vi "Load DB Table.vi"(8 "error in (no error)":errorcluster, 10 "Calibration Mode":bool=TRUE, 11 "ENET in":refnum<class "ENET_BS120x.lvclass">) -> (0 "error out":errorcluster, 3 "ENET out":refnum<class "ENET_BS120x.lvclass">)   [LabVIEW 2021, in "BS120x Driver.lvlib" / "ENET_BS120x.lvclass"]
uses:
  ENET_BS120x.lvclass
  ENET_BS120x.lvclass/ENET_BS120x.ctl
  <resource>/objmgr/xnet.rc
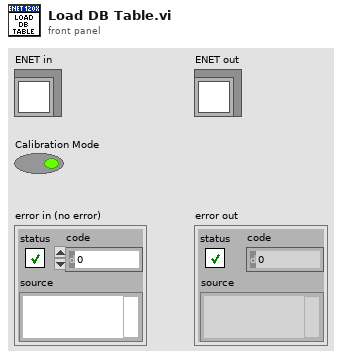
[diagram p1: front panel]
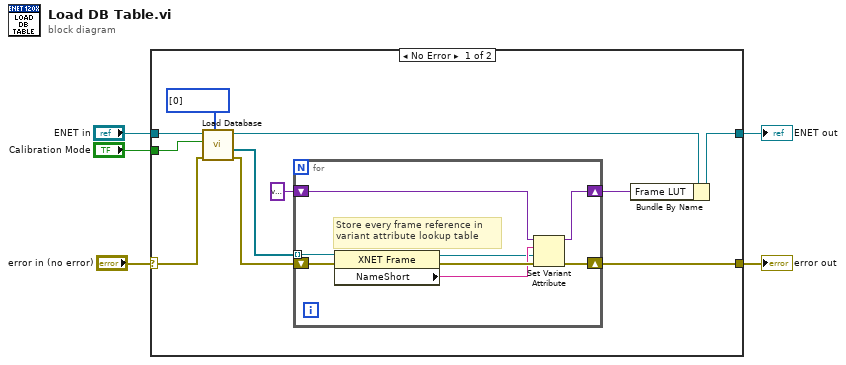
[diagram p0: block diagram]
diagram:
  n1 = case shown="No Error" "error in (no error)" {
    selector: "error in (no error)" -> [w14 w25]
    tunnel: "Calibration Mode" -> [w15 _]
    tunnel: [w13 w25] -> w3
    tunnel: [w11 w26] -> w2
    tunnel: "ENET in" -> [w10 w26]
    frame No Error {
      n2 = call-dynamic "Load Database.vi"("Box ID Array"=u8[] [0], "error in (no error)"=w14, "Calibration Mode"=w15, "Battery Simulator 1200 Driver in"=w10) -> ("error out"=w7:errorcluster, "Specific Frames"=w6:refnum<k21>[], "Battery Simulator 1200 Driver out"=w9:refnum<class "ENET_BS120x.lvclass">)  [unwired: 4 in, 1 out]
      n3 = for {
        shift-right: [w23] -> w12
        shift-left: variant ("Lookup variant") -> [w24]
        shift-right: [w22] -> w13
        shift-left: w7 -> [w20]
        tunnel: w6 -> [w21] mode=indexing
        # "Store every frame reference in variant attribute lookup table"
        n4 = property class="XNET Frame"(reference=w21, error in=w20) -> (reference out=w17:refnum<k21>, error out=w19:errorcluster, "NameShort"=w18:string)
        n5 = Set Variant Attribute(Variant=w24, name=w18, value=w17, error in=w19) -> (Variant out=w23:variant, error out=w22:errorcluster)  [unwired: 1 out]
      }
      n6 = Bundle By Name(cluster=w9, "Frame LUT"=w12) -> (w11:refnum<class "ENET_BS120x.lvclass">)
    }
    frame Error {
    }
  }
  "error out" <- w3
  "ENET out" <- w2
